vi "Init CMY Color.vi"(0 "CMY Color in":refnum<class "CMY Color.lvclass">, 5 "C (0)":u8, 7 "M (0)":u8, 9 "Y (0)":u8, 11 "error in (no error)":errorcluster) -> (4 "CMY Color out":refnum<class "CMY Color.lvclass">, 15 "error out":errorcluster)   [LabVIEW 2018, in "CMY Color.lvclass"]
doc: "Initialize a CMY color"
uses:
  CMY Color.lvclass
  CMY Color.lvclass/CMY Color.ctl
panel:
  # "expressionflow.com"
  # "Copyright (c) 2008 Tomi Maila. All rights reserved."
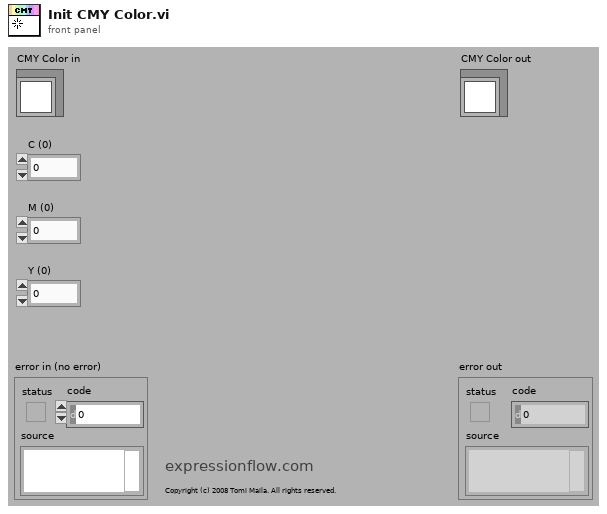
[diagram p1: front panel]
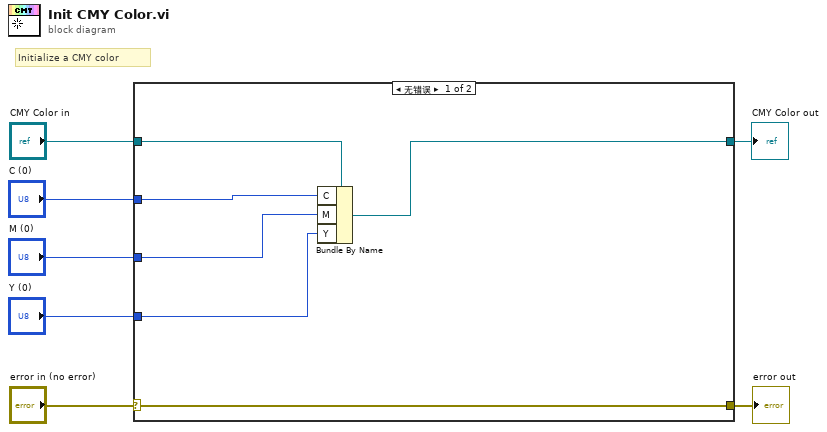
[diagram p0: block diagram]
diagram:
  # "Initialize a CMY color"
  n1 = case shown="无错误" "error in (no error)" {
    selector: "error in (no error)" -> [w13 w15]
    tunnel: [w13 w15] -> w6
    tunnel: [w11 w14] -> w4
    tunnel: "CMY Color in" -> [w12 w14]
    tunnel: "C (0)" -> [w10 _]
    tunnel: "M (0)" -> [w9 _]
    tunnel: "Y (0)" -> [w8 _]
    frame No Error {
      n2 = Bundle By Name(cluster=w12, "C"=w10, "M"=w9, "Y"=w8) -> (w11:refnum<class "CMY Color.lvclass">)
    }
    frame Error {
    }
  }
  "error out" <- w6
  "CMY Color out" <- w4
